vi "BestCamera-position.vi"() -> ()   [LabVIEW 2011]
panel:
  out "Mean":cluster{dbl[], dbl[]}(graph)
  out "Contrast":dbl[](graph)=[0.3193050490763337, 0.30061141956192716, 0.30239991165780683, 0.30047122402971743, 0.2983453929779906, 0.30026280248033993, 0.2948300415387556, 0.3052943699631786, 0.3152640901656084, 0.3581488766839461, 0.3785963254324046, 0.39552770951332494, 0.38705905627433734, 0.40200723872940775, 0.4395993404686244, 0.4426617705097236, 0.43031929209029374, 0.4236369017511004, 0.40177050439420314, 0.37760117109821356, 0.3639153449815441, 0.3597268135868779, 0.3848280287030083, 0.3748641559063438, 0.37703314996300175, 0.3605597635505736, 0.3335687061944306, 0.3115923748332626, 0.2985460236120737, 0.3045024341125598, 0.28980421484286184, 0.2969589065059755, 0.2938250962220528, 0.29954072030737416, 0.29103070633384437]
  out "XY Graph":cluster{dbl[], dbl[]}(graph)
  out "number":dbl=3.77
  in  "file path to tif files with position as name":path=path "C:/temp/z-fokus"
  # "2.345blala.tif"
  # "need till files/stacks in folder like:\n1.23.tif\n2.45.tif\n7.891022.tif\n..."
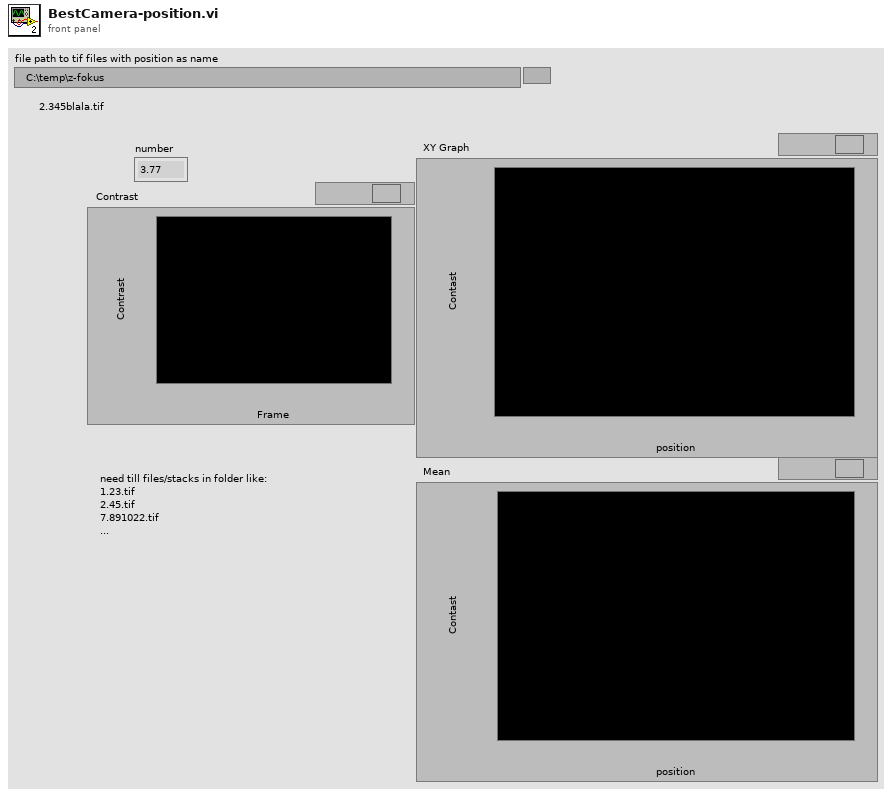
[diagram p1: front panel]
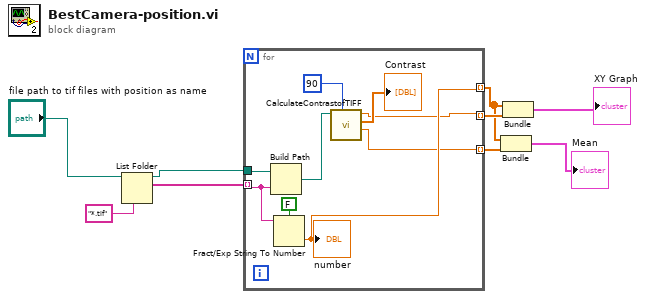
[diagram p0: block diagram]
diagram:
  n1 = List Folder(path="file path to tif files with position as name", pattern="*.tif") -> (path out=w6:path, filenames=w7:string[])  [unwired: 2 in, 2 out]
  n2 = for {
    tunnel: w7 -> [w16] mode=indexing
    tunnel: w6 -> [w18]
    tunnel: [w14] -> w3 mode=indexing
    tunnel: [w11] -> w5 mode=indexing
    tunnel: [w10] -> w4 mode=indexing
    n3 = Build Path(base path=w18, name or relative path=w16) -> (appended path=w17:path)
    n4 = Fract/Exp String To Number(use system decimal point (T)=FALSE, string=w16) -> (number=w14:dbl)  [unwired: 2 in, 1 out]
    "number" <- w14
    n5 = call "CalculateContrastofTIFF.vi"("Offset-Konstante"=i16 90, "file path"=w17) -> ("mean value"=w10:dbl, "Waveform Graph"=→"Contrast":dbl[], "max value"=w11:dbl)  [unwired: 6 in, 1 out]
  }
  n6 = Bundle(w3, w4) -> (→"Mean":cluster{dbl[], dbl[]})  [unwired: 1 in]
  n7 = Bundle(w3, w5) -> (→"XY Graph":cluster{dbl[], dbl[]})  [unwired: 1 in]
